vi "Parse Input String.vi"(7 "delimiter (Tab)":string, 11 "delimited string":string) -> (3 "parsed string":string[][](array[string]))   [LabVIEW 2022 SP3]
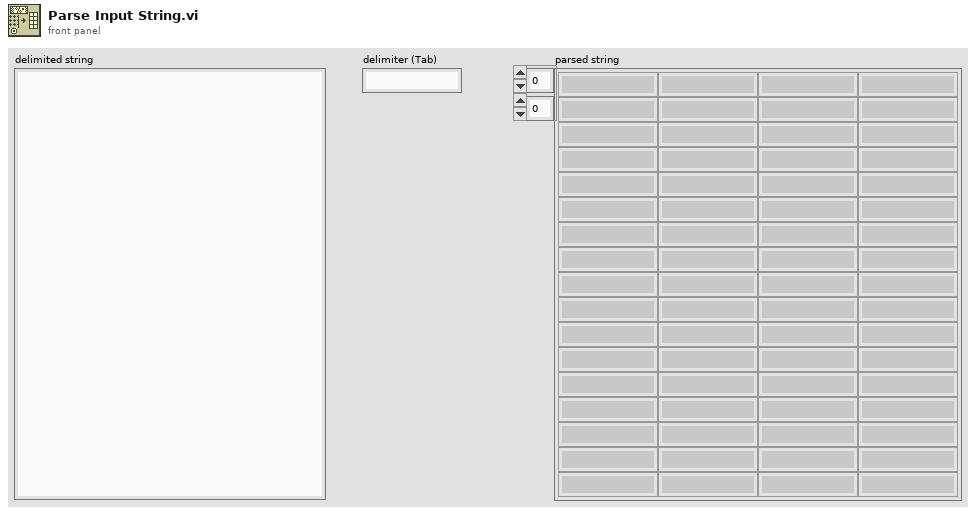
[diagram p1: front panel]
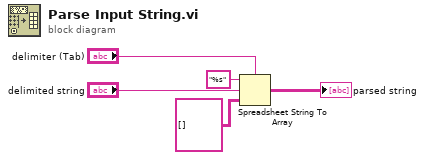
[diagram p0: block diagram]
diagram:
  n1 = Spreadsheet String To Array(delimiter (Tab)="delimiter (Tab)", format string="%s", spreadsheet string="delimited string", array type (2D Dbl)=string[][] []) -> (array=→"parsed string":string[][])
